vi "UI Interlocks.vi"(7 "Menu Ref":refnum<k9>, 8 "error in (no error)":errorcluster, 9 "VI Selected":i32, 11 "New VI Data":T1[](array[typedef])) -> (0 "error out":errorcluster)   [LabVIEW 2023, in "VI Properties Editor.lvlib"]
doc: "Enables or disables several menu items and buttons depending on the state of the system."
uses:
  VI Properties Editor.lvlib
  CTLs/VI Data.ctl
  CTLs/VI Properties.ctl
  <vilib>/picture/picture.llb/imagedata.ctl
  CTLs/Control Properties.ctl
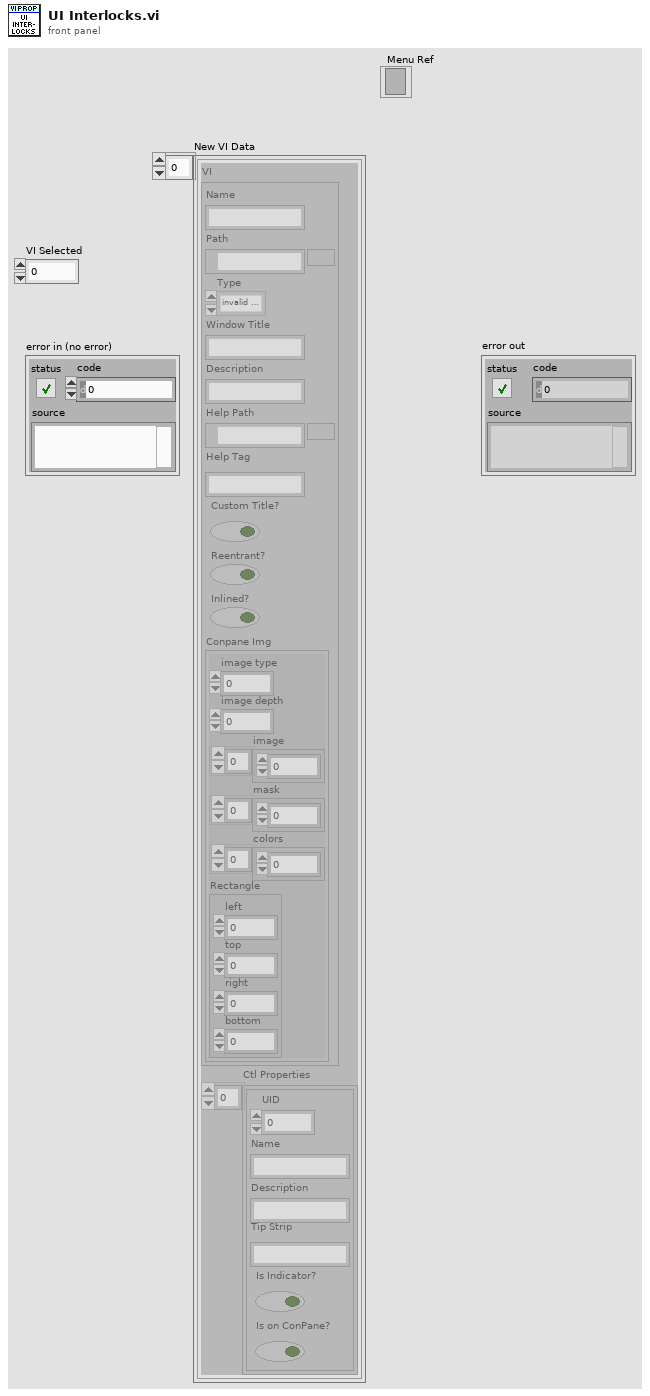
[diagram p1: front panel]
types:
  T1 = typedef "VI Properties Editor.lvlib/VI Data.ctl" = cluster{"VI":T2, "Ctl Properties":T4[]}
  T2 = typedef "VI Properties Editor.lvlib/VI Properties.ctl" = cluster{"Name":string, "Path":path, "Type":enum32{"invalid VI type", "Standard VI", "Control VI", "Global VI", "Polymorphic VI", "Configuration VI", "SubSystem", "Facade VI", "Method VI", "Statechart Diagram VI"}, "Window Title":string, "Description":string, "Help Path":path, "Help Tag":string, "Custom Title?":bool, "Reentrant?":bool, "Inlined?":bool, "Conpane Img":T3}
  T3 = typedef "imagedata.ctl" = cluster{"image type":i32, "image depth":i32, "image":u8[], "mask":u8[], "colors":u32[], "Rectangle":cluster{"left":i16, "top":i16, "right":i16, "bottom":i16}}
  T4 = typedef "VI Properties Editor.lvlib/Control Properties.ctl" = cluster{"UID":i32, "Name":string, "Description":string, "Tip Strip":string, "Is Indicator?":bool, "Is on ConPane?":bool}
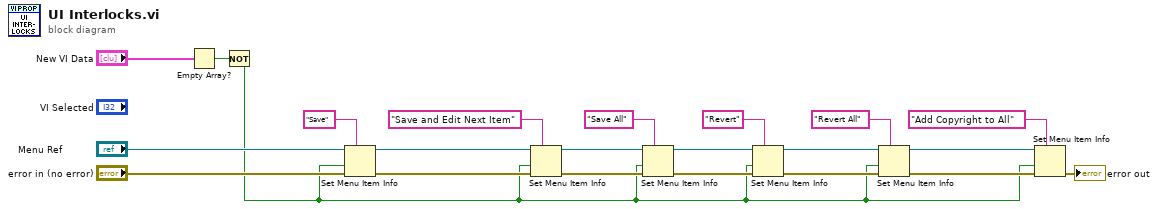
[diagram p0: block diagram]
diagram:
  n1 = Empty Array?(array="New VI Data") -> (empty?=w18:bool)
  n2 = Not(x=w18) -> (.not. x?=w2:bool)
  n3 = Set Menu Item Info(7:"Save" ("item tag"), 8:"error in (no error)", 9:w2, 11:"Menu Ref") -> (0:w14:errorcluster, 3:w15:refnum<k9>)  [unwired: 3 in]
  n4 = Set Menu Item Info(7:"Save and Edit Next Item" ("item tag"), 8:w14, 9:w2, 11:w15) -> (0:w12:errorcluster, 3:w13:refnum<k9>)  [unwired: 3 in]
  n5 = Set Menu Item Info(7:"Save All" ("item tag"), 8:w12, 9:w2, 11:w13) -> (0:w9:errorcluster, 3:w10:refnum<k9>)  [unwired: 3 in]
  n6 = Set Menu Item Info(7:"Revert" ("item tag"), 8:w9, 9:w2, 11:w10) -> (0:w6:errorcluster, 3:w7:refnum<k9>)  [unwired: 3 in]
  n7 = Set Menu Item Info(7:"Revert All" ("item tag"), 8:w6, 9:w2, 11:w7) -> (0:w4:errorcluster, 3:w3:refnum<k9>)  [unwired: 3 in]
  n8 = Set Menu Item Info(7:"Add Copyright to All" ("item tag"), 8:w4, 9:w2, 11:w3) -> (0:→"error out":errorcluster)  [unwired: 3 in, 1 out]
